vi "PI_Feedforward.vi"(5 "Motor Effort Axis":dbl[](array[numeric]) format="%_6g", 6 "dT":dbl, 7 "Position Axis":dbl[](array[numeric]) format="%_6g", 9 "Control Inputs":T2={"Kp"=0.01, "Ki"=0.0, "i upper"=0.0, "i lower"=0.0, "Output upper"=1.0, "Output lower"=-1.0}, 10 "Feed Back":dbl, 11 "Target":dbl) -> (1 "Term Indicators":T1, 2 "Output":dbl, 3 "Error":dbl)   [LabVIEW 2016]
uses:
  <vilib>/gmath/NI_Gmath.lvlib
  <vilib>/Rock Robotics/WPI/ThirdParty/CanMotor/TalonSRX/WPI_CANTalonSRX_APIFeedbackSelect.ctl
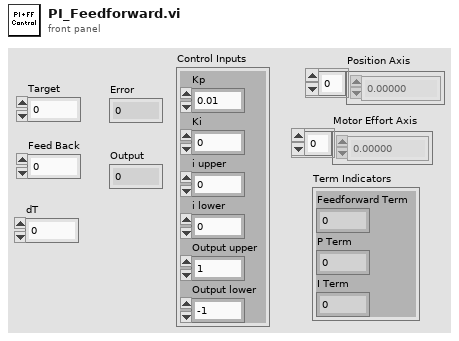
[diagram p1: front panel]
types:
  T1 = cluster{"Feedforward Term":dbl, "P Term ":dbl, "I Term":dbl}
  T2 = cluster{"Kp":dbl, "Ki":dbl, "i upper":dbl, "i lower":dbl, "Output upper":dbl, "Output lower":dbl}
  T3 = typedef "WPI_CANTalonSRX_APIFeedbackSelect.ctl" = enum16{"Digital Quadrature Encoder", "Analog Potentiometer", "Analog Encoder", "Count on Quad-A (Rising-Edge)", "Count on Quad-A (Falling-Edge)", "CTR Magnetic Enc (Absolute)", "CTR Magnetic Enc (Relative)", "Pulse Width"}
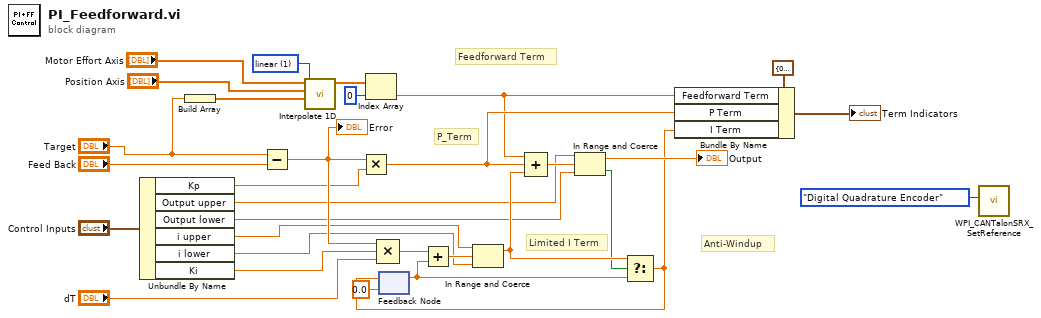
[diagram p0: block diagram]
diagram:
  w15 = 1 items=["nearest", "linear", "spline", "cubic Hermite", "Lagrange"] ("method")
  # "Feedforward Term"
  # "Anti-Windup"
  # "Limited I Term"
  # "P_Term"
  n1 = Unbundle By Name("Control Inputs") -> ("Kp"=w21:dbl, "Output upper"=w20:dbl, "Output lower"=w19:dbl, "i upper"=w18:dbl, "i lower"=w17:dbl, "Ki"=w16:dbl)
  n2 = Build Array("Target") -> (w13:dbl[])
  n3 = Subtract(x="Target", y="Feed Back") -> (x-y=w31:dbl)
  "Error" <- w31
  n4 = call <vilib>:"Interpolate 1D.vi"("method"=w15, "xi"=w13, "X"="Position Axis", "Y"="Motor Effort Axis") -> ("yi"=w10:dbl[])  [unwired: 5 in, 2 out]
  n5 = Multiply(x=w31, y=w21) -> (x*y=w6:dbl)
  n6 = Index Array(array=w10, index=0) -> (element=w4:dbl)
  n7 = Compound Arithmetic op=MULTIPLY(w31, w16, "dT") -> (w29:dbl)
  n8 = feedback #1(0.0 ("i upper")) -> (w24:dbl)
  n9 = Add(x=w29, y=w24) -> (x+y=w28:dbl)
  n10 = In Range and Coerce(upper limit=w18, x=w28, lower limit=w17) -> (coerced(x)=w25:dbl)  [unwired: 1 out]
  n11 = Compound Arithmetic op=ADD(w4, w6, w25) -> (w27:dbl)
  n12 = In Range and Coerce(upper limit=w20, x=w27, lower limit=w19) -> (coerced(x)=→"Output":dbl, In Range?=w23:bool)
  n13 = Select(t=w25, s=w23, f=w24) -> (s? t:f=w5:dbl)
  n14 = feedback-in #1(w5) -> ()
  n15 = Bundle By Name(cluster=T1 {"Feedforward Term"=0.0, "P Term "=0.0, "I Term"=0.0} ("Term Indicators"), "Feedforward Term"=w4, "P Term"=w6, "I Term"=w5) -> (→"Term Indicators":T1)
  n16 = call <vilib>:"WPI_CANTalonSRX_SetReference.vi"("Feedback Reference"=WPI_CANTalonSRX_APIFeedbackSelect."Digital Quadrature Encoder") -> ("error in (no error)"=w1:errorcluster)  [unwired: 8 in, 2 out]
